vi "LS336_RampStatus_DP_ver1.0.vi"(0 "GPIB ADR (18)":i16=18, 1 "Output's control loop (1)":i32=1, 2 "Mode: (default: 2)":i16(ring)=2 items=["Do nothing to mark the end of the transfer", "Send NL (linefeed) with EOI after the data bytes.", "Send EOI with the last data byte in the string(default)"], 3 "error in":errorcluster) -> (4 "Ramping On?":bool, 5 "Ramping Active?":bool, 6 "dump GPIB ADR":i16, 7 "Ramp Rate":dbl, 8 "Ramp Rate":string, 9 "error out":errorcluster)   [LabVIEW 2012]
doc: "This VI returns the status of the setpoint ramp function. The Model 336 can generate a smooth setpoint ramp when the setpoint units are expressed in temperature. Once the ramping feature is turned on, its action is initiated by a setpoint change. When a new setpoint is entered, the instrument changes the setpoint temperature from the old value to the new value at the ramp rate. The Setpoint Ramping function applies to the Heater Outputs (1 and 2) only."
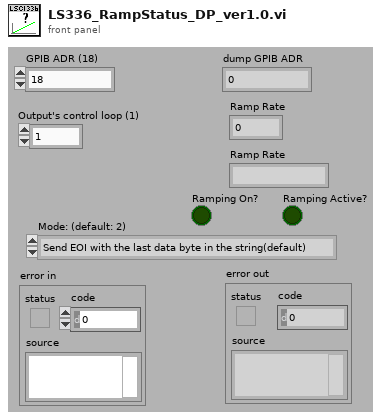
[diagram p1: front panel]
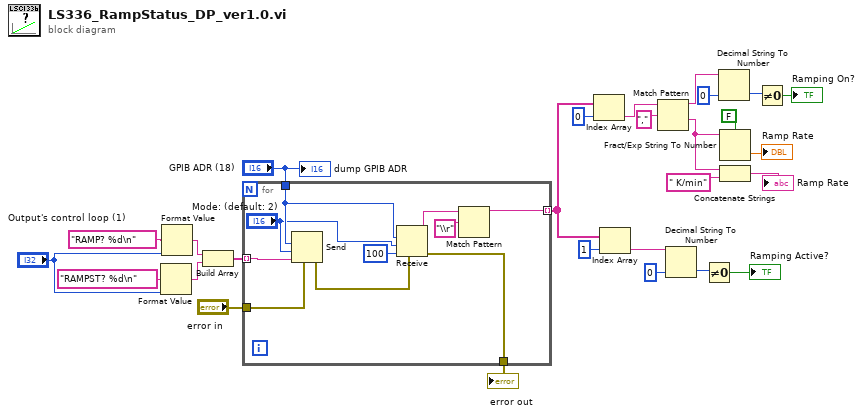
[diagram p0: block diagram]
diagram:
  n1 = Format Value(format string="RAMPST? %d\n", value (0)="Output's control loop (1)") -> (output string=w23:string)  [unwired: 1 out]
  n2 = Format Value(format string="RAMP? %d\n", value (0)="Output's control loop (1)") -> (output string=w24:string)  [unwired: 1 out]
  n3 = Build Array(w24, w23) -> (w22:string[])
  n4 = for {
    tunnel: w22 -> [w36] mode=indexing
    tunnel: "error in" -> [w35]
    tunnel: [w33] -> w20
    tunnel: "GPIB ADR (18)" -> [w32]
    tunnel: [w28] -> w6 mode=indexing
    n5 = Send(2:w32, 3:"Mode: (default: 2)", 4:w35, 5:w36) -> (8:w34:errorcluster)  [unwired: 1 in, 2 out]
    n6 = Receive(4:w34, 6:100 ("count"), 7:"Mode: (default: 2)", 8:w32) -> (0:w33:errorcluster, 3:w30:string)  [unwired: 3 out]
    n7 = Match Pattern(string=w30, regular expression="\\r") -> (before substring=w28:string)  [unwired: 4 out]
  }
  "error out" <- w20
  n8 = Index Array(array=w6, index=0) -> (element=w17:string)
  n9 = Index Array(array=w6, index=1) -> (element=w3:string)
  n10 = Match Pattern(string=w17, regular expression=",") -> (before substring=w16:string, after substring=w10:string)  [unwired: 3 out]
  n11 = Decimal String To Number(string=w3, default (0L)=0 ("default (0 I32)")) -> (number=w4:i32)  [unwired: 2 out]
  n12 = Not Equal To 0?(x=w4) -> (x != 0?=→"Ramping Active?":bool)
  n13 = Decimal String To Number(string=w16, default (0L)=0 ("default (0 I32)")) -> (number=w14:i32)  [unwired: 2 out]
  n14 = Fract/Exp String To Number(use system decimal point (T)=FALSE, string=w10) -> (number=→"Ramp Rate":dbl)  [unwired: 3 out]
  n15 = Concatenate Strings(w10, " K/min" ("string")) -> (→"Ramp Rate":string)
  n16 = Not Equal To 0?(x=w14) -> (x != 0?=→"Ramping On?":bool)
  "dump GPIB ADR" <- "GPIB ADR (18)"
